vi "PackWay.vi"(10 "FileLen":u32) -> (0 "I-1024包数":u32, 1 "I-128包数":u32, 2 "帧包方式":enum16{"128K", "1024K-128K"}(ring), 3 "帧数":u32)   [LabVIEW 2013]
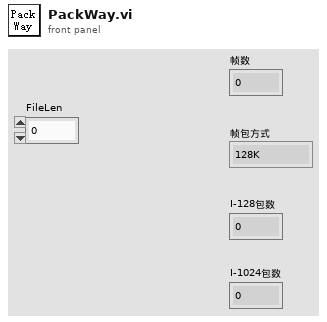
[diagram p1: front panel]
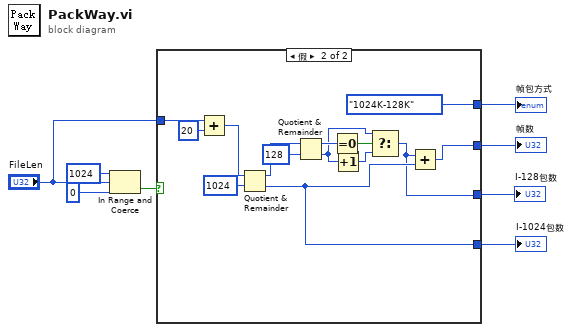
[diagram p0: block diagram]
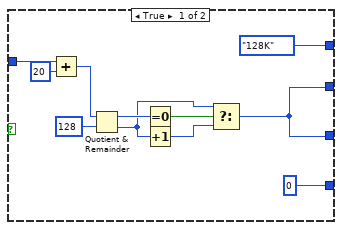
[diagram p2: hidden frame]
diagram:
  n1 = In Range and Coerce(upper limit=1024, x="FileLen", lower limit=0) -> (In Range?=w6:bool)  [unwired: 1 out]
  n2 = case shown="假" w6 {
    tunnel: [enum16{"128K", "1024K-128K"}."128K" ("帧包方式") enum16{"128K", "1024K-128K"}."1024K-128K" ("帧包方式")] -> w5
    tunnel: "FileLen" -> [w18 w32]
    tunnel: [w9 w26] -> w3
    tunnel: [u32 0 w21] -> w2
    tunnel: [w9 w20] -> w1
    frame True {
      n3 = Add(x=w18, y=20) -> (x+y=w16:u32)
      n4 = Quotient & Remainder(x=w16, y=128) -> (x-y*floor(x/y)=w14:u32, floor(x/y)=w11:u32)
      n5 = Equal To 0?(x=w14) -> (x = 0?=w13:bool)
      n6 = Increment(x=w11) -> (x+1=w12:u32)
      n7 = Select(t=w11, s=w13, f=w12) -> (s? t:f=w9:u32)
    }
    frame False {
      n8 = Add(x=w32, y=20) -> (x+y=w30:u32)
      n9 = Quotient & Remainder(x=w30, y=1024) -> (x-y*floor(x/y)=w28:u32, floor(x/y)=w21:u32)
      n10 = Quotient & Remainder(x=w28, y=128) -> (x-y*floor(x/y)=w25:u32, floor(x/y)=w22:u32)
      n11 = Equal To 0?(x=w25) -> (x = 0?=w24:bool)
      n12 = Increment(x=w22) -> (x+1=w23:u32)
      n13 = Select(t=w22, s=w24, f=w23) -> (s? t:f=w20:u32)
      n14 = Add(x=w20, y=w21) -> (x+y=w26:u32)
    }
  }
  "帧数" <- w3
  "帧包方式" <- w5
  "I-128包数" <- w1
  "I-1024包数" <- w2
